vi "Логи_UKF.vi"() -> ()   [LabVIEW 2013]
panel:
  in  "Tab Control":T1(tab)
  out "pos":cluster{dbl[], dbl[]}[](graph)
  out "pos 2":cluster{dbl[], dbl[]}[](graph)
  out "vel":cluster{dbl[], dbl[]}[](graph)
  out "bias":cluster{dbl[], dbl[]}[](graph)
  out "angle":cluster{dbl[], dbl[]}[](graph)
  out "ID параметров":u8[](array[numeric])
  out "Длина заголовка":i32
  out "Заголовок":string
  out "Количество параметров":u8
  out "size (in bytes)":i64
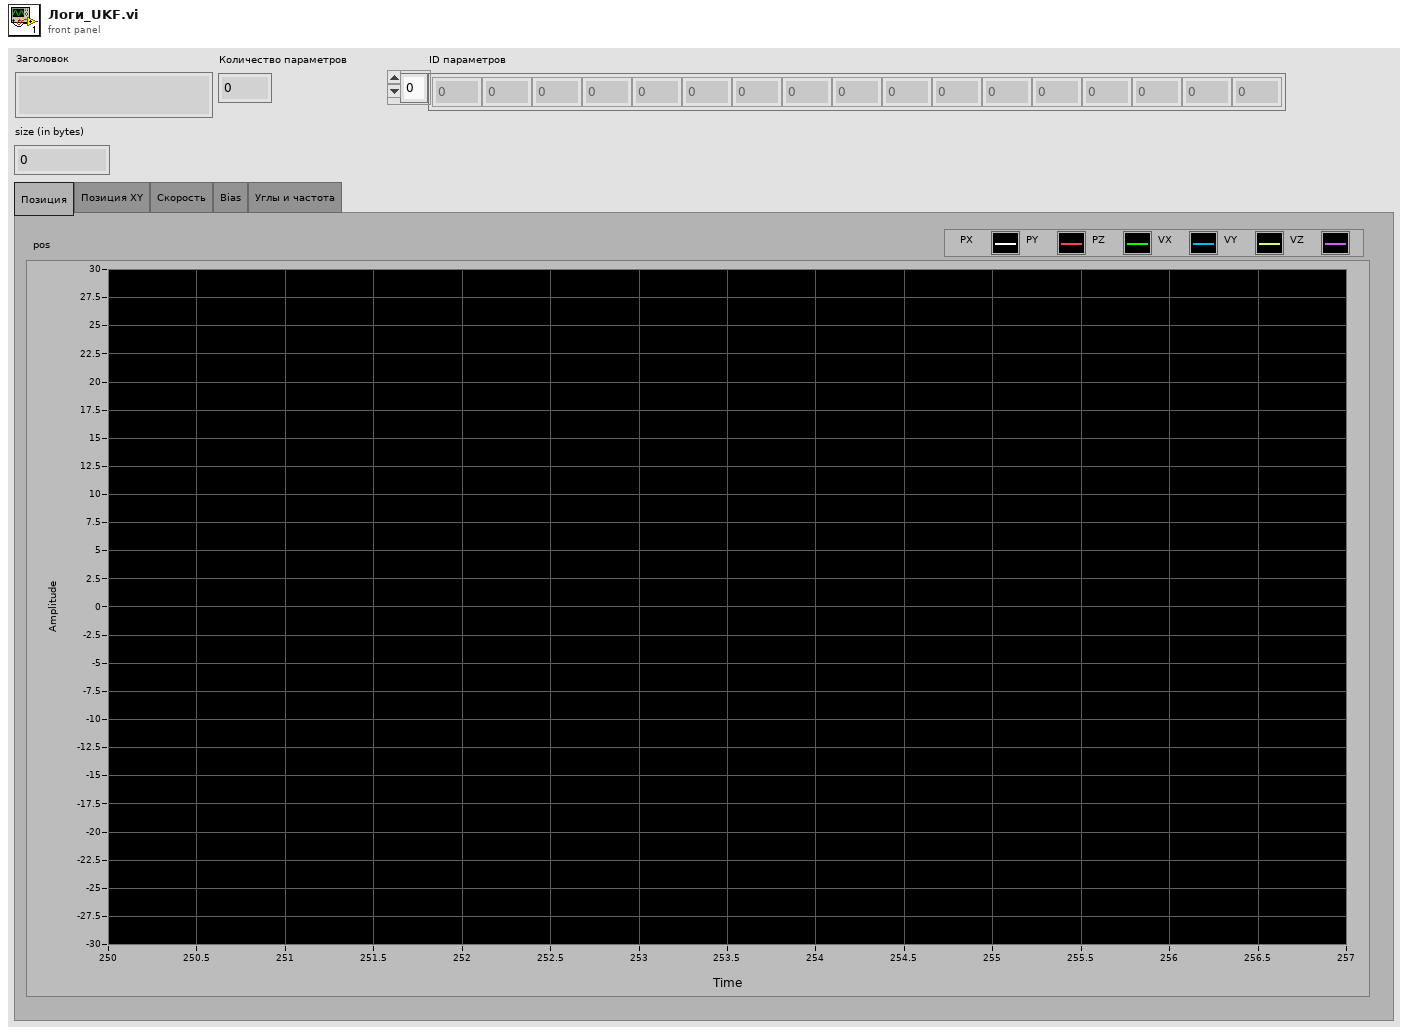
[diagram p1: front panel]
types:
  T1 = enum32{"Позиция", "Позиция XY", "Скорость", "Bias", "Углы и частота"}
  T2 = enum16{"open", "replace", "create", "open or create", "replace or create", "replace or create with confirmation"}
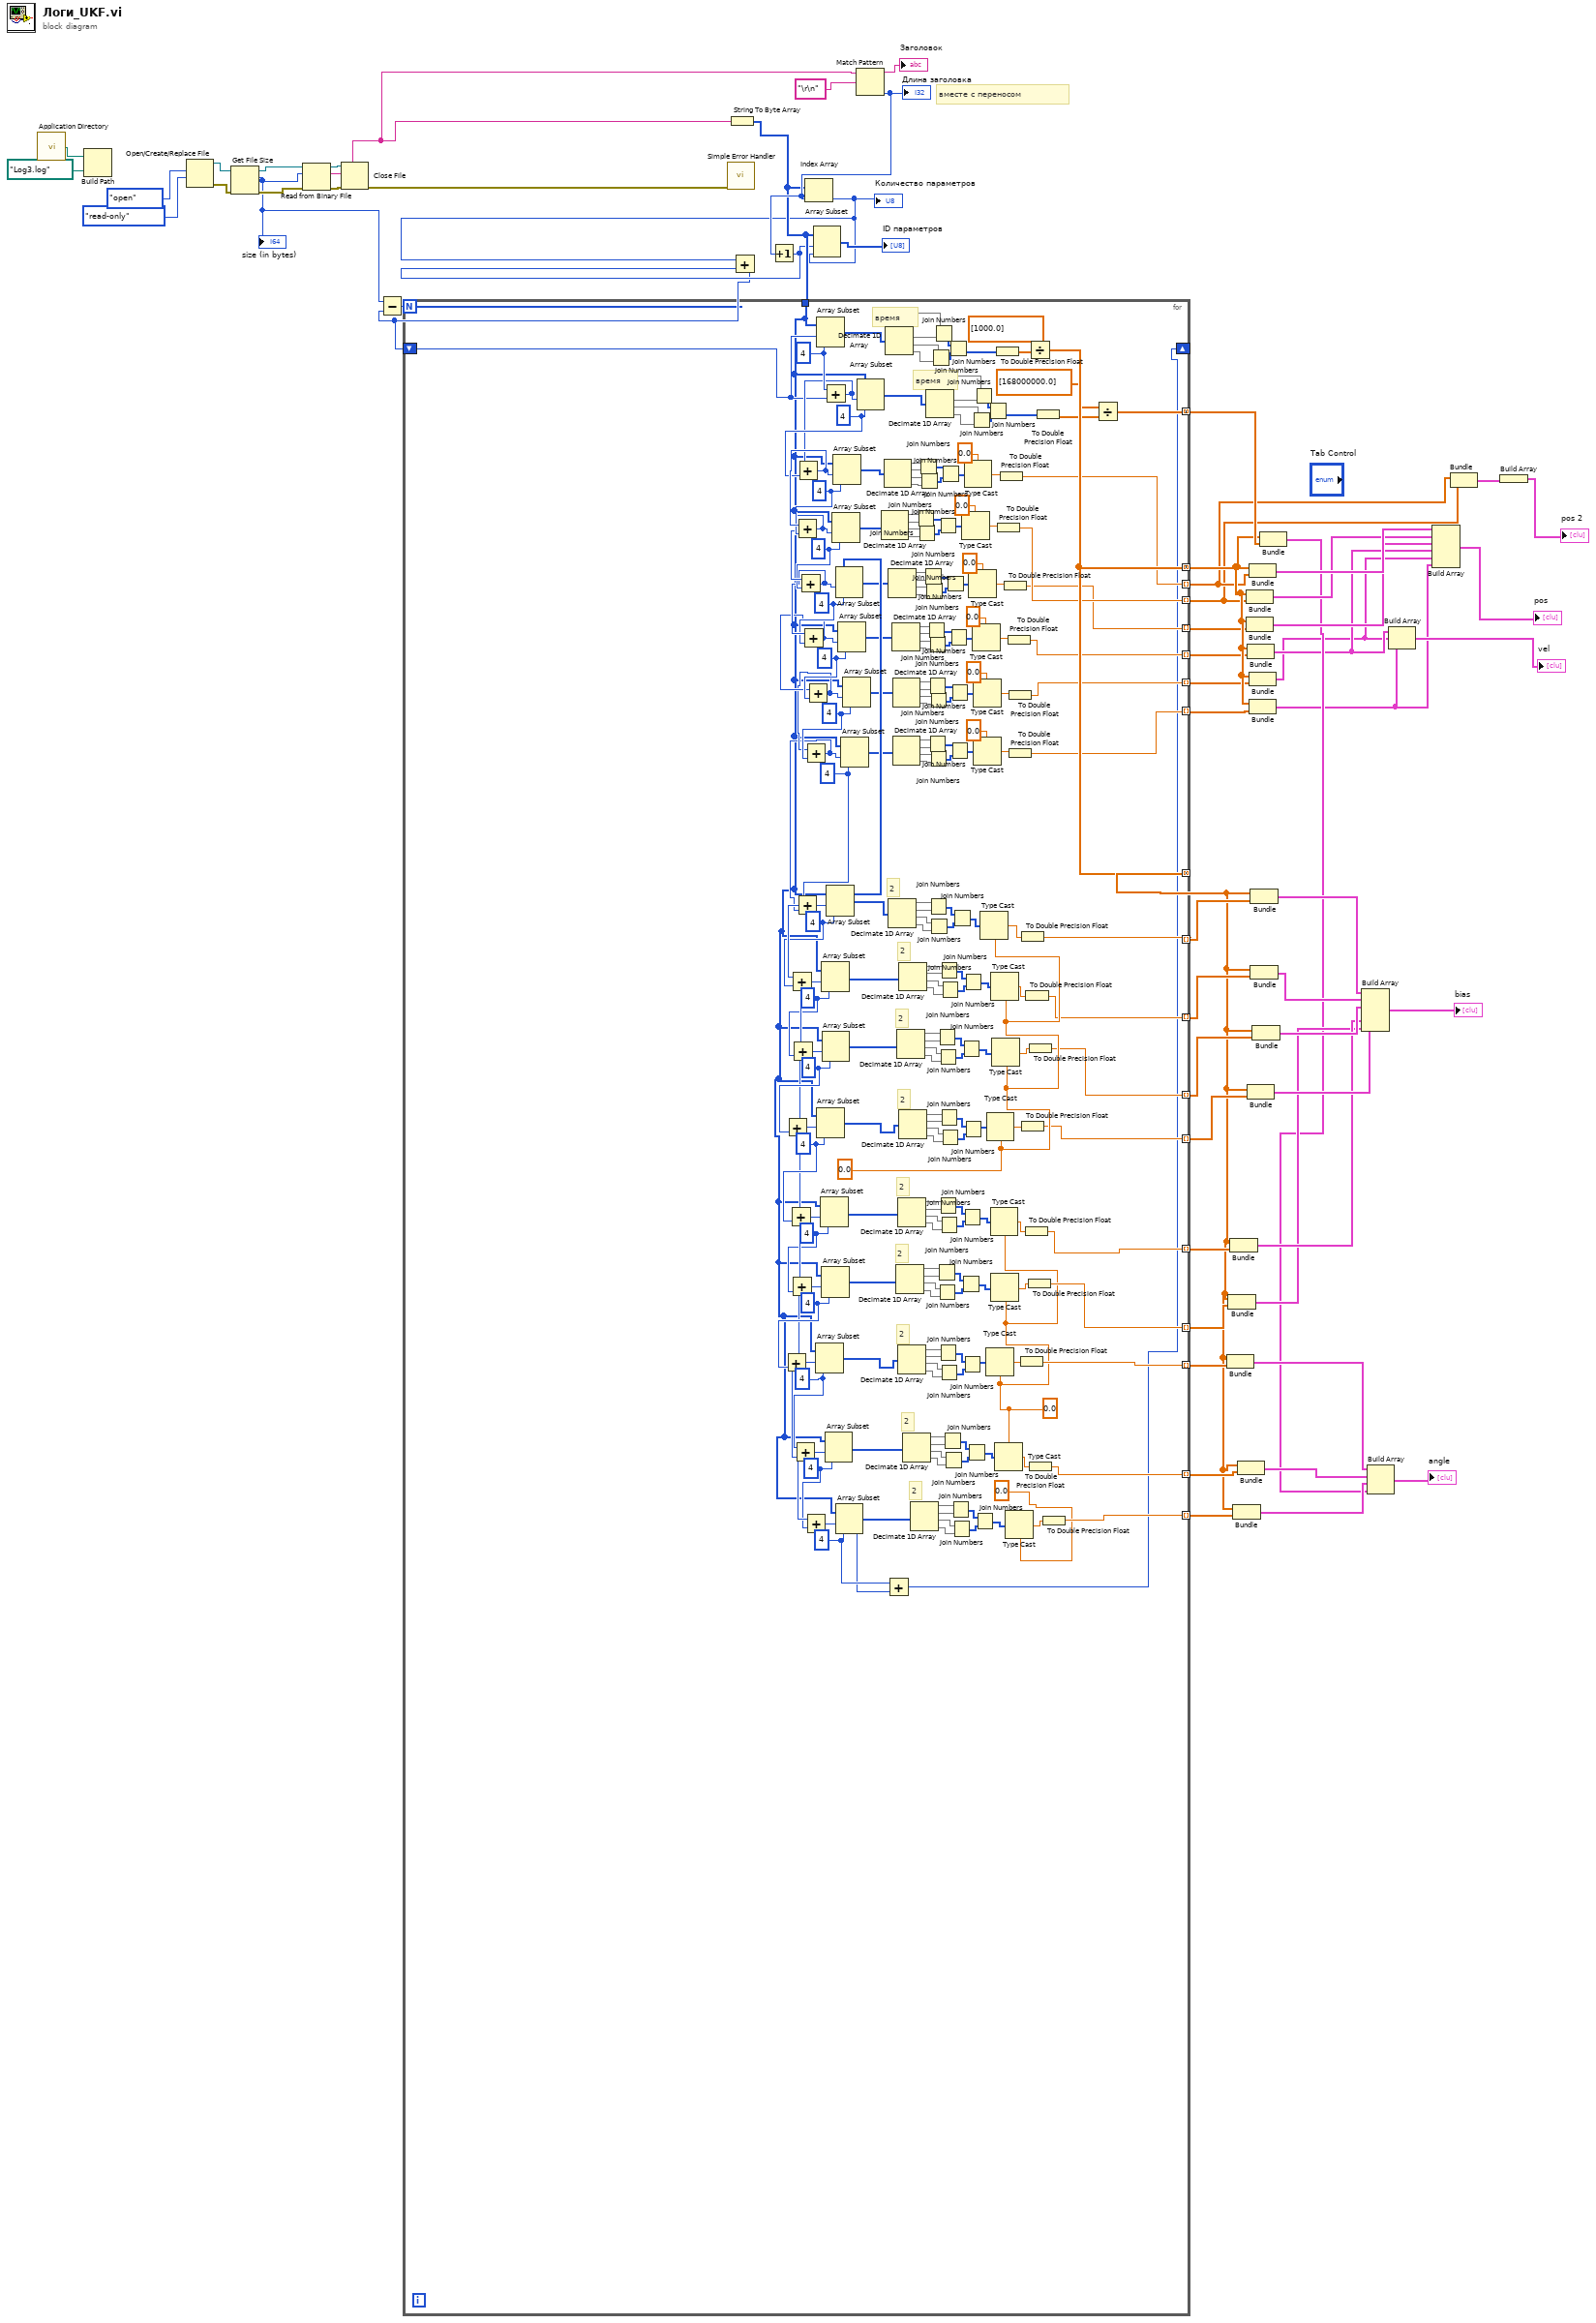
[diagram p0: block diagram]
diagram:
  # "вместе с переносом"
  n1 = call <vilib>:"Application Directory.vi"() -> ("Application Directory"=w59:path)
  n2 = Build Path(base path=w59, name or relative path=path "Log3.log" ("default name")) -> ()  [unwired: 1 out]
  n3 = Open/Create/Replace File(operation (0:open)=T2."open", access (0:read/write)=enum16{"read/write", "read-only", "write-only"}."read-only") -> (refnum out=w56:refnum<file>, error out=w54:errorcluster)  [unwired: 4 in, 1 out]
  n4 = Get File Size(file=w56, error in=w54) -> (refnum out=w55:refnum<file>, size (in bytes)=w46:i64, 0:w53:errorcluster)
  "size (in bytes)" <- w46
  n5 = Read from Binary File(8:w53, 10:w46, 11:w55) -> (0:w57:errorcluster, 2:w52:string, 3:w58:refnum<file>)  [unwired: 3 in, 1 out]
  n6 = Close File(refnum=w58, error in=w57) -> (error out=w62:errorcluster)  [unwired: 1 out]
  n7 = call <vilib>:"Simple Error Handler.vi"("error in (no error)"=w62) -> ()  [unwired: 4 in, 5 out]
  n8 = String To Byte Array(string=w52) -> (unsigned byte array=w47:u8[])
  n9 = Match Pattern(string=w52, regular expression="\r\n" ("format string")) -> (before substring=→"Заголовок":string, offset past match=w49:i32)  [unwired: 1 in, 2 out]
  "Длина заголовка" <- w49
  n10 = Increment(x=w49) -> (x+1=w44:i32)
  n11 = Index Array(array=w47, index=w49) -> (element=w45:u8)
  "Количество параметров" <- w45
  n12 = Add(x=w45, y=w44) -> (x+y=w43:i32)
  n13 = Subtract(x=w46, y=w43) -> (x-y=w42:i64)
  n14 = for {
    N: w42 -> [_]
    tunnel: w47 -> [w133]
    shift-right: [w63] -> _
    shift-left: w43 -> [w141]
    tunnel: [w220] -> w24 mode=concatenating
    tunnel: [w165] -> w27 mode=indexing
    tunnel: [w164] -> w28 mode=indexing
    tunnel: [w163] -> w29 mode=indexing
    tunnel: [w162] -> w30 mode=indexing
    tunnel: [w220] -> w35 mode=concatenating
    tunnel: [w182] -> w39 mode=indexing
    tunnel: [w181] -> w38 mode=indexing
    tunnel: [w180] -> w37 mode=indexing
    tunnel: [w166] -> w36 mode=concatenating
    tunnel: [w135] -> w26 mode=indexing
    tunnel: [w134] -> w25 mode=indexing
    tunnel: [w71] -> w4 mode=indexing
    tunnel: [w70] -> w3 mode=indexing
    tunnel: [w69] -> w23 mode=indexing
    tunnel: [w68] -> w22 mode=indexing
    tunnel: [w67] -> w21 mode=indexing
    tunnel: [w66] -> w20 mode=indexing
    w65 = 4 ("length")
    w160 = 4 ("length")
    w170 = 4 ("length")
    w138 = sgl 0.0
    w137 = 4 ("length")
    w215 = 4 ("length")
    w213 = 4 ("length")
    w140 = 4 ("length")
    w218 = 4 ("length")
    w219 = 4 ("length")
    w221 = 4 ("length")
    w223 = 4 ("length")
    w225 = 4 ("length")
    w229 = sgl 0.0
    w184 = 4 ("length")
    w277 = 4 ("length")
    w275 = 4 ("length")
    w278 = 4 ("length")
    w171 = 4 ("length")
    # "2"
    # "2"
    # "время"
    # "2"
    # "2"
    # "2"
    # "2"
    # "2"
    # "2"
    # "2"
    # "время"
    n15 = Array Subset(array=w133, index=w141, length=w171) -> (w264:u8[])
    n16 = Add(x=w171, y=w141) -> (x+y=w169:i32)
    n17 = Add(x=w169, y=w170) -> (x+y=w226:i32)
    n18 = Add(x=w226, y=w225) -> (x+y=w224:i32)
    n19 = Add(x=w224, y=w223) -> (x+y=w222:i32)
    n20 = Add(x=w222, y=w221) -> (x+y=w217:i32)
    n21 = Add(x=w217, y=w219) -> (x+y=w216:i32)
    n22 = Add(x=w216, y=w218) -> (x+y=w139:i32)
    n23 = Add(x=w140, y=w139) -> (x+y=w279:i32)
    n24 = Add(x=w279, y=w278) -> (x+y=w276:i32)
    n25 = Add(x=w276, y=w275) -> (x+y=w274:i32)
    n26 = Add(x=w274, y=w277) -> (x+y=w183:i32)
    n27 = Add(x=w183, y=w184) -> (x+y=w214:i32)
    n28 = Add(x=w214, y=w213) -> (x+y=w212:i32)
    n29 = Add(x=w212, y=w215) -> (x+y=w136:i32)
    n30 = Add(x=w137, y=w136) -> (x+y=w161:i32)
    n31 = Add(x=w161, y=w160) -> (x+y=w64:i32)
    n32 = Array Subset(array=w133, index=w136, length=w137) -> (w191:u8[])
    n33 = Array Subset(array=w133, index=w183, length=w184) -> (w237:u8[])
    n34 = Array Subset(array=w133, index=w214, length=w213) -> (w205:u8[])
    n35 = Array Subset(array=w133, index=w276, length=w275) -> (w251:u8[])
    n36 = Array Subset(array=w133, index=w212, length=w215) -> (w198:u8[])
    n37 = Array Subset(array=w133, index=w274, length=w277) -> (w244:u8[])
    n38 = Array Subset(array=w133, index=w161, length=w160) -> (w153:u8[])
    n39 = Array Subset(array=w133, index=w279, length=w278) -> (w265:u8[])
    n40 = Array Subset(array=w133, index=w224, length=w223) -> (w76:u8[])
    n41 = Array Subset(array=w133, index=w226, length=w225) -> (w123:u8[])
    n42 = Array Subset(array=w133, index=w222, length=w221) -> (w75:u8[])
    n43 = Array Subset(array=w133, index=w64, length=w65) -> (w146:u8[])
    n44 = Array Subset(array=w133, index=w217, length=w219) -> (w74:u8[])
    n45 = Array Subset(array=w133, index=w139, length=w140) -> (w72:u8[])
    n46 = Array Subset(array=w133, index=w216, length=w218) -> (w73:u8[])
    n47 = Array Subset(array=w133, index=w169, length=w170) -> (w173:u8[])
    n48 = Decimate 1D Array(w76) -> (w120:u8[], w121:u8[], w119:u8[], w118:u8[])
    n49 = Decimate 1D Array(w123) -> (w130:u8[], w131:u8[], w129:u8[], w128:u8[])
    n50 = Add(x=w65, y=w64) -> (x+y=w63:i32)
    n51 = Decimate 1D Array(w264) -> (w267:u8[], w268:u8[], w269:u8[], w270:u8[])
    n52 = Decimate 1D Array(w75) -> (w111:u8[], w112:u8[], w110:u8[], w109:u8[])
    n53 = Decimate 1D Array(w265) -> (w272:u8[], w273:u8[], w261:u8[], w260:u8[])
    n54 = Decimate 1D Array(w74) -> (w102:u8[], w103:u8[], w101:u8[], w100:u8[])
    n55 = Decimate 1D Array(w73) -> (w93:u8[], w94:u8[], w92:u8[], w91:u8[])
    n56 = Decimate 1D Array(w72) -> (w84:u8[], w85:u8[], w83:u8[], w82:u8[])
    n57 = Decimate 1D Array(w198) -> (w203:u8[], w204:u8[], w202:u8[], w201:u8[])
    n58 = Decimate 1D Array(w244) -> (w249:u8[], w250:u8[], w248:u8[], w247:u8[])
    n59 = Decimate 1D Array(w205) -> (w210:u8[], w211:u8[], w209:u8[], w208:u8[])
    n60 = Decimate 1D Array(w191) -> (w196:u8[], w197:u8[], w195:u8[], w194:u8[])
    n61 = Decimate 1D Array(w251) -> (w256:u8[], w257:u8[], w255:u8[], w254:u8[])
    n62 = Decimate 1D Array(w237) -> (w242:u8[], w243:u8[], w241:u8[], w240:u8[])
    n63 = Decimate 1D Array(w153) -> (w158:u8[], w159:u8[], w157:u8[], w156:u8[])
    n64 = Decimate 1D Array(w146) -> (w151:u8[], w152:u8[], w150:u8[], w149:u8[])
    n65 = Join Numbers(hi=w120, lo=w121) -> ((hi.lo)=w117:u16[])
    n66 = Join Numbers(hi=w119, lo=w118) -> ((hi.lo)=w116:u16[])
    n67 = Join Numbers(hi=w130, lo=w131) -> ((hi.lo)=w127:u16[])
    n68 = Join Numbers(hi=w129, lo=w128) -> ((hi.lo)=w126:u16[])
    n69 = Join Numbers(hi=w111, lo=w112) -> ((hi.lo)=w108:u16[])
    n70 = Join Numbers(hi=w110, lo=w109) -> ((hi.lo)=w107:u16[])
    n71 = Join Numbers(hi=w102, lo=w103) -> ((hi.lo)=w99:u16[])
    n72 = Join Numbers(hi=w101, lo=w100) -> ((hi.lo)=w98:u16[])
    n73 = Join Numbers(hi=w93, lo=w94) -> ((hi.lo)=w90:u16[])
    n74 = Join Numbers(hi=w84, lo=w85) -> ((hi.lo)=w81:u16[])
    n75 = Join Numbers(hi=w92, lo=w91) -> ((hi.lo)=w89:u16[])
    n76 = Join Numbers(hi=w83, lo=w82) -> ((hi.lo)=w80:u16[])
    n77 = Join Numbers(hi=w272, lo=w273) -> ((hi.lo)=w259:u16[])
    n78 = Decimate 1D Array(w173) -> (w175:u8[], w176:u8[], w177:u8[], w178:u8[])
    n79 = Join Numbers(hi=w261, lo=w260) -> ((hi.lo)=w258:u16[])
    n80 = Join Numbers(hi=w269, lo=w270) -> ((hi.lo)=w266:u16[])
    n81 = Join Numbers(hi=w267, lo=w268) -> ((hi.lo)=w271:u16[])
    n82 = Join Numbers(hi=w203, lo=w204) -> ((hi.lo)=w200:u16[])
    n83 = Join Numbers(hi=w249, lo=w250) -> ((hi.lo)=w246:u16[])
    n84 = Join Numbers(hi=w202, lo=w201) -> ((hi.lo)=w199:u16[])
    n85 = Join Numbers(hi=w117, lo=w116) -> ((hi.lo)=w115:u32[])
    n86 = Join Numbers(hi=w248, lo=w247) -> ((hi.lo)=w245:u16[])
    n87 = Join Numbers(hi=w210, lo=w211) -> ((hi.lo)=w207:u16[])
    n88 = Join Numbers(hi=w196, lo=w197) -> ((hi.lo)=w193:u16[])
    n89 = Join Numbers(hi=w256, lo=w257) -> ((hi.lo)=w253:u16[])
    n90 = Join Numbers(hi=w242, lo=w243) -> ((hi.lo)=w239:u16[])
    n91 = Join Numbers(hi=w209, lo=w208) -> ((hi.lo)=w206:u16[])
    n92 = Join Numbers(hi=w195, lo=w194) -> ((hi.lo)=w192:u16[])
    n93 = Join Numbers(hi=w255, lo=w254) -> ((hi.lo)=w252:u16[])
    n94 = Join Numbers(hi=w241, lo=w240) -> ((hi.lo)=w238:u16[])
    n95 = Join Numbers(hi=w127, lo=w126) -> ((hi.lo)=w125:u32[])
    n96 = Join Numbers(hi=w158, lo=w159) -> ((hi.lo)=w155:u16[])
    n97 = Join Numbers(hi=w157, lo=w156) -> ((hi.lo)=w154:u16[])
    n98 = Join Numbers(hi=w108, lo=w107) -> ((hi.lo)=w106:u32[])
    n99 = Join Numbers(hi=w271, lo=w266) -> ((hi.lo)=w232:u32[])
    n100 = Join Numbers(hi=w99, lo=w98) -> ((hi.lo)=w97:u32[])
    n101 = Join Numbers(hi=w90, lo=w89) -> ((hi.lo)=w88:u32[])
    n102 = Join Numbers(hi=w81, lo=w80) -> ((hi.lo)=w79:u32[])
    n103 = Join Numbers(hi=w151, lo=w152) -> ((hi.lo)=w148:u16[])
    n104 = Join Numbers(hi=w150, lo=w149) -> ((hi.lo)=w147:u16[])
    n105 = Join Numbers(hi=w259, lo=w258) -> ((hi.lo)=w228:u32[])
    n106 = Join Numbers(hi=w200, lo=w199) -> ((hi.lo)=w188:u32[])
    n107 = Join Numbers(hi=w246, lo=w245) -> ((hi.lo)=w234:u32[])
    n108 = Join Numbers(hi=w207, lo=w206) -> ((hi.lo)=w186:u32[])
    n109 = Join Numbers(hi=w193, lo=w192) -> ((hi.lo)=w189:u32[])
    n110 = Join Numbers(hi=w253, lo=w252) -> ((hi.lo)=w231:u32[])
    n111 = Join Numbers(hi=w239, lo=w238) -> ((hi.lo)=w235:u32[])
    n112 = Type Cast(type=sgl 0.0, x=w115) -> (*(type *) &x=w114:sgl)
    n113 = Join Numbers(hi=w155, lo=w154) -> ((hi.lo)=w143:u32[])
    n114 = Type Cast(type=sgl 0.0, x=w125) -> (*(type *) &x=w124:sgl)
    n115 = Join Numbers(hi=w177, lo=w178) -> ((hi.lo)=w174:u16[])
    n116 = Type Cast(type=sgl 0.0, x=w106) -> (*(type *) &x=w105:sgl)
    n117 = Join Numbers(hi=w175, lo=w176) -> ((hi.lo)=w179:u16[])
    n118 = Join Numbers(hi=w148, lo=w147) -> ((hi.lo)=w145:u32[])
    n119 = Type Cast(type=sgl 0.0, x=w97) -> (*(type *) &x=w96:sgl)
    n120 = Type Cast(type=sgl 0.0, x=w88) -> (*(type *) &x=w87:sgl)
    n121 = Type Cast(type=sgl 0.0, x=w79) -> (*(type *) &x=w78:sgl)
    n122 = Type Cast(type=w229, x=w228) -> (*(type *) &x=w227:sgl)
    n123 = Join Numbers(hi=w179, lo=w174) -> ((hi.lo)=w172:u32[])
    n124 = Type Cast(type=w138, x=w189) -> (*(type *) &x=w190:sgl)
    n125 = Type Cast(type=w229, x=w235) -> (*(type *) &x=w236:sgl)
    n126 = Type Cast(type=w138, x=w186) -> (*(type *) &x=w185:sgl)
    n127 = Type Cast(type=w229, x=w231) -> (*(type *) &x=w230:sgl)
    n128 = Type Cast(type=w138, x=w188) -> (*(type *) &x=w187:sgl)
    n129 = Type Cast(type=w229, x=w234) -> (*(type *) &x=w233:sgl)
    n130 = To Double Precision Float(number=w232) -> (double precision float=w263:dbl[])
    n131 = To Double Precision Float(number=w114) -> (double precision float=w70:dbl)
    n132 = Type Cast(type=w138, x=w143) -> (*(type *) &x=w142:sgl)
    n133 = To Double Precision Float(number=w124) -> (double precision float=w71:dbl)
    n134 = To Double Precision Float(number=w105) -> (double precision float=w69:dbl)
    n135 = To Double Precision Float(number=w96) -> (double precision float=w68:dbl)
    n136 = Type Cast(type=sgl 0.0, x=w145) -> (*(type *) &x=w144:sgl)
    n137 = To Double Precision Float(number=w87) -> (double precision float=w67:dbl)
    n138 = To Double Precision Float(number=w78) -> (double precision float=w66:dbl)
    n139 = To Double Precision Float(number=w190) -> (double precision float=w180:dbl)
    n140 = To Double Precision Float(number=w227) -> (double precision float=w165:dbl)
    n141 = To Double Precision Float(number=w236) -> (double precision float=w162:dbl)
    n142 = To Double Precision Float(number=w185) -> (double precision float=w182:dbl)
    n143 = To Double Precision Float(number=w230) -> (double precision float=w164:dbl)
    n144 = Divide(x=w263, y=dbl[] [1000.0]) -> (x/y=w220:dbl[])
    n145 = To Double Precision Float(number=w187) -> (double precision float=w181:dbl)
    n146 = To Double Precision Float(number=w233) -> (double precision float=w163:dbl)
    n147 = To Double Precision Float(number=w142) -> (double precision float=w135:dbl)
    n148 = To Double Precision Float(number=w172) -> (double precision float=w168:dbl[])
    n149 = To Double Precision Float(number=w144) -> (double precision float=w134:dbl)
    n150 = Divide(x=dbl[] [168000000.0] ("y"), y=w168) -> (x/y=w166:dbl[])
  }
  n151 = Array Subset(array=w47, index=w44, length=w45) -> (→"ID параметров":u8[])
  n152 = Bundle(w24, w37) -> (w11:cluster{dbl[], dbl[]})  [unwired: 1 in]
  n153 = Bundle(w24, w38) -> (w14:cluster{dbl[], dbl[]})  [unwired: 1 in]
  n154 = Bundle(w24, w39) -> (w15:cluster{dbl[], dbl[]})  [unwired: 1 in]
  n155 = Bundle(w24, w25) -> (w9:cluster{dbl[], dbl[]})  [unwired: 1 in]
  n156 = Bundle(w24, w26) -> (w10:cluster{dbl[], dbl[]})  [unwired: 1 in]
  n157 = Bundle(w35, w3) -> (w18:cluster{dbl[], dbl[]})  [unwired: 1 in]
  n158 = Bundle(w35, w23) -> (w17:cluster{dbl[], dbl[]})  [unwired: 1 in]
  n159 = Bundle(w35, w22) -> (w7:cluster{dbl[], dbl[]})  [unwired: 1 in]
  n160 = Bundle(w24, w30) -> (w31:cluster{dbl[], dbl[]})  [unwired: 1 in]
  n161 = Bundle(w35, w4) -> (w19:cluster{dbl[], dbl[]})  [unwired: 1 in]
  n162 = Bundle(w35, w21) -> (w6:cluster{dbl[], dbl[]})  [unwired: 1 in]
  n163 = Bundle(w35, w20) -> (w5:cluster{dbl[], dbl[]})  [unwired: 1 in]
  n164 = Bundle(w24, w27) -> (w34:cluster{dbl[], dbl[]})  [unwired: 1 in]
  n165 = Bundle(w24, w28) -> (w33:cluster{dbl[], dbl[]})  [unwired: 1 in]
  n166 = Bundle(w24, w29) -> (w32:cluster{dbl[], dbl[]})  [unwired: 1 in]
  n167 = Bundle(w35, w36) -> (w8:cluster{dbl[], dbl[]})  [unwired: 1 in]
  n168 = Build Array(w34, w33, w32, w31, w15, w14) -> (→"bias":cluster{dbl[], dbl[]}[])
  n169 = Build Array(w11, w10, w9, w8) -> (→"angle":cluster{dbl[], dbl[]}[])
  n170 = Build Array(w7, w6, w5) -> (→"vel":cluster{dbl[], dbl[]}[])
  n171 = Build Array(w19, w18, w17, w7, w6, w5) -> (→"pos":cluster{dbl[], dbl[]}[])
  n172 = Bundle(w4, w3) -> (w2:cluster{dbl[], dbl[]})  [unwired: 1 in]
  n173 = Build Array(w2) -> (→"pos 2":cluster{dbl[], dbl[]}[])
